vi "DIO-449 Read Industrial Port PointbyPoint.vi"() -> ()   [LabVIEW 8.6]
uses:
  <vilib>/UeiDaq/UeiDaqConfigureTimingForSimpleIO.vi
  <vilib>/UeiDaq/UeiDaqReadOneDigitalScanUInt16.vi
  <vilib>/UeiDaq/UeiDaqCreateAISession.vi
  <libdir>/resource/objmgr/UeiDaq.rc
  <vilib>/UeiDaq/UeiDaqReadOneDigitalScanUInt32.vi
  <vilib>/UeiDaq/UeiDaqCreateDIIndustrialSession.vi
  <vilib>/UeiDaq/UeiDaqReadOneScaledScan.vi
panel:
  in  "AC mode":i32
  in  "high threshold":dbl
  in  "low threshold":dbl
  in  "gain":i32
  in  "High Threshold":dbl[](array[numeric])
  in  "Low Threshold":dbl[](array[numeric])
  out "Voltage measured at each input line 2":dbl[](array[numeric]) format="%.2f"
  in  "Mux":i32[](array[ring]) items=["Disconnected", "Pull-Up", "Diagnostic"]
  in  "AC mode":i32[](array[numeric])
  in  "Gain":i32[](array[numeric])
  in  "Voltage Supply":dbl[](array[numeric])
  out "Voltage measured at each input line":dbl[](array[numeric]) format="%.2f"
  in  "AI Resource":string
  in  "Digital filter min.\ninput width (ms)":dbl
  out "device name":string
  out "DI Resolution (bits)":u32
  out "Raw Data":i32[](array[numeric]) format="%x"
  out "DO ports":bool[][](array[boolean])
  in  "DI Resource":string
  out "Total scans acquired":u32
  in  "Refresh rate (ms)":u32
  in  "stop":bool
  # "DIO-449 READ FROM DIGITAL IN (Point by Point)"
  # "1/ Set the resource name -->"
  # "2/ Set the input port parameters -->"
  # "3/ Set the update rate -->"
  # "Pull-up mux not an option"
  # "Sets high and low threshold\nfor all 48 channels"
  # "To switch to line level mode use \"diline\" as subsystem name\n\nFor example:\npdna://192.168.100.2/dev0/diline0:47 gives independent access to all 48 inputs\n\npdna://192.168.100.2/dev0/di0,1 gives access to the 48 inputs in 2 banks of 24 lines."
  # "if wired, will set high and\nlow thresholds, gain and \nAC mode to unique values for individual channels"
  # "0 - gain  1 /range +/-215"
  # "1 - gain  2 /range +/-107"
  # "------------>"
  # "2 - gain  5 /range +/-42"
  # "3 - gain 10/range +/-21"
  # "23"
  # "22"
  # "21"
  # "20"
  # "19"
  # "18"
  # "17"
  # "16"
  # "15"
  # "14"
  # "13"
  # "12"
  # "11"
  # "10"
  # "9"
  # "8"
  # "7"
  # "6"
  # "5"
  # "4"
  # "3"
  # "2"
  # "1"
  # "0"
  # "47"
  # "46"
  # "45"
  # "44"
  # "43"
  # "42"
  # "41"
  # "40"
  # "39"
  # "38"
  # "37"
  # "36"
  # "35"
  # "34"
  # "33"
  # "32"
  # "31"
  # "30"
  # "29"
  # "28"
  # "27"
  # "26"
  # "25"
  # "24"
  # "0"
  # "1"
  # "2"
  # "3"
  # "4"
  # "5"
  # "6"
  # "7"
  # "8"
  # "9"
  # "10"
  # "11"
  # "12"
  # "13"
  # "14"
  # "15"
  # "16"
  # "17"
  # "18"
  # "19"
  # "20"
  # "21"
  # "22"
  # "23"
  # "24"
  # "25"
  # "26"
  # "27"
  # "28"
  # "29"
  # "30"
  # "31"
  # "32"
  # "33"
  # "34"
  # "35"
  # "36"
  # "37"
  # "38"
  # "39"
  # "40"
  # "41"
  # "42"
  # "43"
  # "44"
  # "45"
  # "46"
  # "47"
  # "Device info"
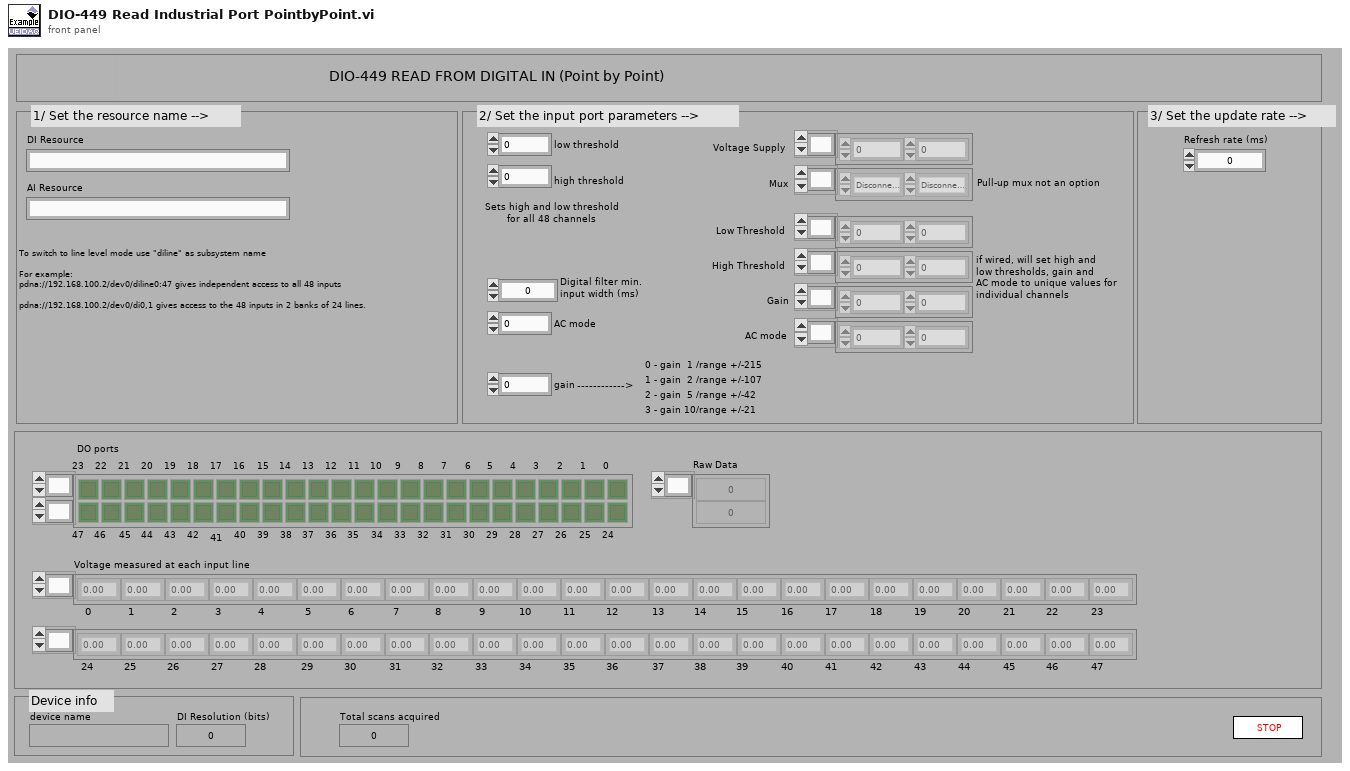
[diagram p1: front panel]
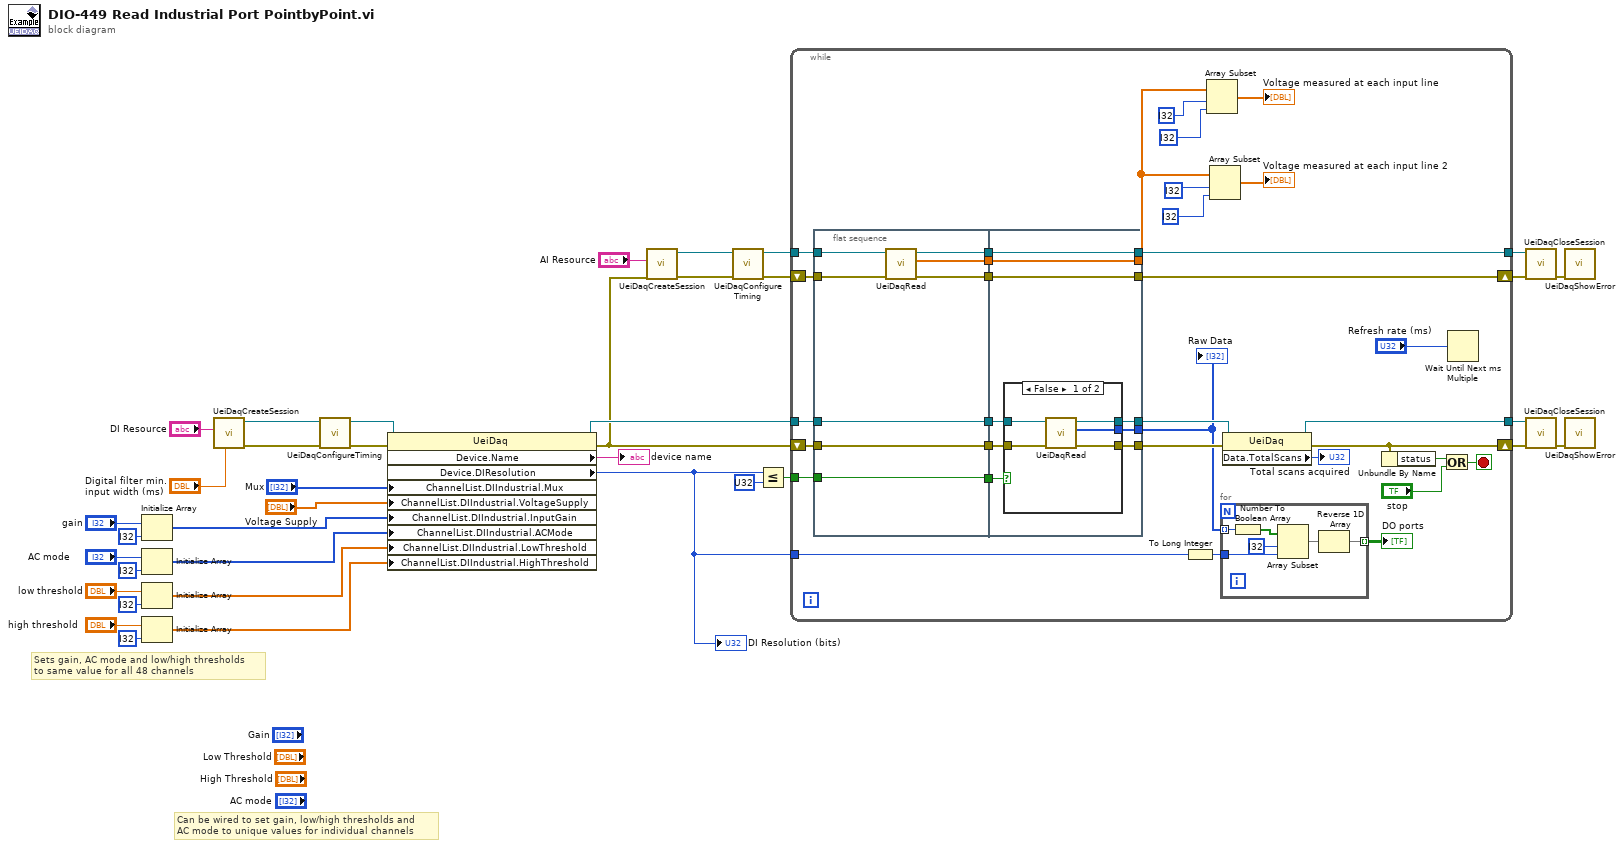
[diagram p0: block diagram]
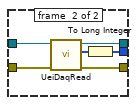
[diagram p2: hidden frame]
diagram:
  # "Sets gain, AC mode and low/high thresholds\nto same value for all 48 channels"
  # "Can be wired to set gain, low/high thresholds and\nAC mode to unique values for individual channels"
  n1 = Initialize Array("gain", i32 ? ("dimension size")) -> (w1:i32[])
  n2 = Initialize Array("AC mode", i32 ? ("dimension size")) -> (w4:i32[])
  n3 = Initialize Array("low threshold", i32 ? ("dimension size")) -> (w3:dbl[])
  n4 = Initialize Array("high threshold", i32 ? ("dimension size")) -> (w2:dbl[])
  n5 = call-poly <vilib>:"UeiDaqCreateSession.vi"("Minimum pulse width"="Digital filter min.\ninput width (ms)", "Resource"="DI Resource") -> ("error out"=w35:errorcluster, "UeiDaq Refnum Out"=w36:refnum<k20>)  [unwired: 4 in, 4 out]
  n6 = call-poly <vilib>:"UeiDaqConfigureTiming.vi"("error in (no error)"=w35, "UeiDaq Refnum In"=w36) -> ("error out"=w31:errorcluster, "UeiDaq Refnum Out"=w33:refnum<k20>)  [unwired: 1 in, 7 out]
  n7 = property class="UeiDaq"(reference=w33, error in=w31, "ChannelList.DIIndustrial.Mux"="Mux", "ChannelList.DIIndustrial.VoltageSupply"="Voltage Supply", "ChannelList.DIIndustrial.InputGain"=w1, "ChannelList.DIIndustrial.ACMode"=w4, "ChannelList.DIIndustrial.LowThreshold"=w3, "ChannelList.DIIndustrial.HighThreshold"=w2) -> (reference out=w32:refnum<k20>, error out=w20:errorcluster, "Device.Name"=→"device name":string, "Device.DIResolution"=w26:u32)
  "DI Resolution (bits)" <- w26
  n8 = call-poly <vilib>:"UeiDaqCreateSession.vi"("error in (no error)"=w20, "Resource"="AI Resource") -> ("error out"=w21:errorcluster, "UeiDaq Refnum Out"=w22:refnum<k20>)  [unwired: 4 in, 4 out]
  n9 = call-poly <vilib>:"UeiDaqConfigureTiming.vi"("error in (no error)"=w21, "UeiDaq Refnum In"=w22) -> ("error out"=w18:errorcluster, "UeiDaq Refnum Out"=w19:refnum<k20>)  [unwired: 1 in, 7 out]
  n10 = Less Or Equal?(x=w26, y=u32 ?) -> (x <= y?=w29:bool)
  n11 = while {
    tunnel: w32 -> [w67]
    tunnel: w29 -> [w69]
    tunnel: [w65] -> w27
    tunnel: w26 -> [w58]
    tunnel: w19 -> [w56]
    tunnel: [w54] -> w17
    shift-right: [w53] -> w16
    shift-left: w18 -> [w55]
    shift-right: [w60] -> w28
    shift-left: w20 -> [w68]
    stop <- w59 stop-if-true
    n12 = flat-sequence {
      tunnel: w69 -> [w71]
      tunnel: w68 -> [w72]
      tunnel: w67 -> [w73]
      tunnel: w56 -> [w78]
      tunnel: w55 -> [w77]
      tunnel: [w72] -> w51
      tunnel: [w73] -> w50
      tunnel: [w76] -> w49
      tunnel: [w75] -> w48
      tunnel: [w74] -> w47
      tunnel: [w71] -> w46
      tunnel: [w85] -> w41
      tunnel: [w86] -> w53
      tunnel: [w87] -> w54
      tunnel: [w80] -> w64
      tunnel: [w81] -> w66
      tunnel: w51 -> [w83]
      tunnel: w50 -> [w82]
      tunnel: w49 -> [w87]
      tunnel: w48 -> [w86]
      tunnel: w47 -> [w85]
      tunnel: w46 -> [w84]
      tunnel: [w79] -> w45
      frame #0 {
        n13 = call-poly <vilib>:"UeiDaqRead.vi"("error in (no error)"=w77, "UeiDaq Refnum In"=w78) -> ("error out"=w75:errorcluster, "Scaled Data"=w74:dbl[], "UeiDaq Refnum Out"=w76:refnum<k20>)  [unwired: 7 out]
      }
      frame #1 {
        n14 = case shown="False" w84 {
          tunnel: [w92 w97] -> w81
          tunnel: [w91 w96] -> w80
          tunnel: [w90 w95] -> w79
          tunnel: w83 -> [w88 w93]
          tunnel: w82 -> [w89 w94]
          frame #0 {
            n15 = call-poly <vilib>:"UeiDaqRead.vi"("error in (no error)"=w88, "UeiDaq Refnum In"=w89) -> ("error out"=w92:errorcluster, "Raw Data"=w90:i32[], "UeiDaq Refnum Out"=w91:refnum<k20>)  [unwired: 7 out]
          }
          frame #1 {
            n16 = call-poly <vilib>:"UeiDaqRead.vi"("error in (no error)"=w93, "UeiDaq Refnum In"=w94) -> ("error out"=w97:errorcluster, "Raw Data"=w98:i16[], "UeiDaq Refnum Out"=w96:refnum<k20>)  [unwired: 7 out]
            n17 = To Long Integer(number=w98) -> (32bit integer=w95:i32[])
          }
        }
      }
    }
    n18 = To Long Integer(number=w58) -> (32bit integer=w52:i32)
    n19 = Array Subset(array=w41, index=i32 ?, length=i32 ?) -> (→"Voltage measured at each input line":dbl[])
    n20 = Array Subset(array=w41, index=i32 ?, length=i32 ?) -> (→"Voltage measured at each input line 2":dbl[])
    n21 = for {
      tunnel: w45 -> [w104] mode=indexing
      tunnel: w52 -> [w101]
      tunnel: [w99] -> w57 mode=indexing
      n22 = Number To Boolean Array(number=w104) -> (Boolean array=w103:bool[])
      n23 = Array Subset(array=w103, index=i32 ?, length=w101) -> (w100:bool[])
      n24 = Reverse 1D Array(array=w100) -> (reversed array=w99:bool[])
    }
    "DO ports" <- w57
    n25 = property class="UeiDaq"(reference=w64, error in=w66) -> (reference out=w65:refnum<k20>, error out=w60:errorcluster, "Data.TotalScans"=→"Total scans acquired":u32)
    n26 = Unbundle By Name(w60) -> ("status"=w62:bool)
    n27 = Or(x=w62, y="stop") -> (x .or. y?=w59:bool)
    n28 = Wait Until Next ms Multiple(millisecond multiple="Refresh rate (ms)") -> ()  [unwired: 1 out]
    "Raw Data" <- w45
  }
  n29 = call <vilib>:"UeiDaqCloseSession.vi"("error in (no error)"=w16, "UeiDaq Refnum In"=w17) -> ("error out"=w15:errorcluster)  [unwired: 1 in, 8 out]
  n30 = call <vilib>:"UeiDaqCloseSession.vi"("error in (no error)"=w28, "UeiDaq Refnum In"=w27) -> ("error out"=w37:errorcluster)  [unwired: 1 in, 8 out]
  n31 = call <vilib>:"UeiDaqShowError.vi"("error in (no error)"=w15) -> ()  [unwired: 1 in, 10 out]
  n32 = call <vilib>:"UeiDaqShowError.vi"("error in (no error)"=w37) -> ()  [unwired: 1 in, 10 out]
